vi "ClearResources.vi"() -> ()   [LabVIEW 2020, in "AIM664LV.lvlib"]
uses:
  AIM664LV.lvlib
panel:
  out "resources":T1(array[cluster])
  out "error out":errorcluster
  out "NuOfServers":u32
  out "size(s)":i32
  out "Array":errorcluster[](array[cluster])
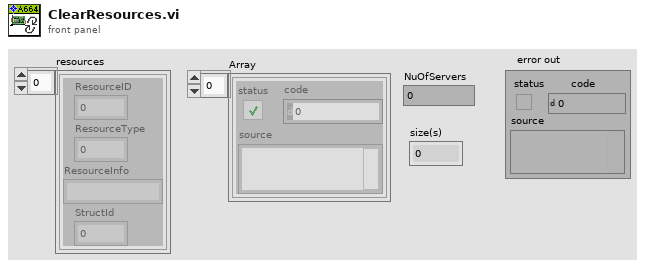
[diagram p1: front panel]
types:
  T1 = cluster{"ResourceID":u32, "ResourceType":u32, "ResourceInfo":string, "StructId":u32}[]
  T2 = cluster{"ResourceID":u32, "ResourceType":u32, "ResourceInfo":string, "StructId":u32}
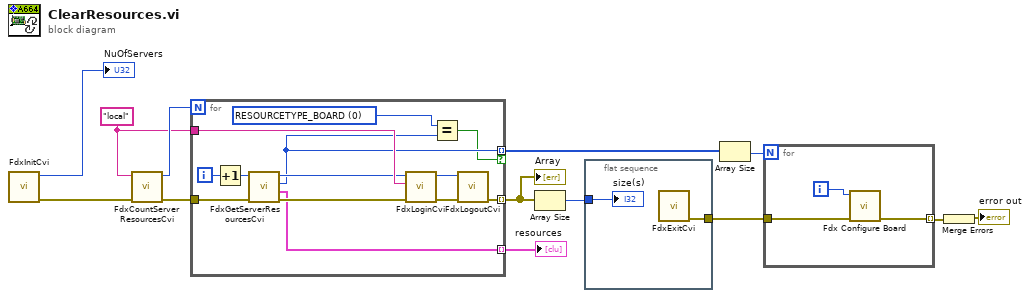
[diagram p0: block diagram]
diagram:
  w6 = "local" ("SrvName(local)")
  n1 = call "FdxInitCvi.vi"() -> ("error out"=w9:errorcluster, "Number of Servers"=→"NuOfServers":u32)  [unwired: 10 in]
  n2 = call "FdxCountServerResourcesCvi.vi"("error in"=w9, "SrvName (local)"=w6) -> ("error out"=w12:errorcluster, "Number of Resources"=w13:u32)  [unwired: 8 in]
  n3 = for {
    N: w13 -> [_]
    tunnel: w12 -> [w26]
    tunnel: [w20] -> w11 mode=indexing
    tunnel: [w19] -> w7 mode=indexing
    tunnel: w6 -> [w18]
    tunnel: [w15] -> w5 mode=indexing if=w14
    i -> [w25]
    w16 = u32 0 items=["RESOURCETYPE_BOARD"=0, "RESOURCETYPE_PORT"=1, "RESOURCETYPE_ALL"=20] ("ResourceType")
    n4 = Increment(x=w25) -> (x+1=w24:i32)
    n5 = call "FdxGetServerResourcesCvi.vi"("error in"=w26, "ServerRElement"=w24) -> ("error out"=w23:errorcluster, "ServerResourceInfo"=w19:T2, "ResourceType"=w15:u32, "Resource ID"=w17:u32)  [unwired: 4 in, 2 out]
    n6 = call "FdxLoginCvi.vi"("error in"=w23, "SrvName"=w18, "ResourceID"=w17) -> ("error out"=w22:errorcluster, "InstrumentHandle"=w21:u32)  [unwired: 7 in]
    n7 = Equal?(x=w16, y=w15) -> (x = y?=w14:bool)
    n8 = call "FdxLogoutCvi.vi"("error in"=w22, "InstrumentHandle"=w21) -> ("error out"=w20:errorcluster)  [unwired: 9 in]
  }
  "Array" <- w11
  "resources" <- w7
  n9 = Array Size(array=w11) -> (size(s)=w10:i32)
  n10 = flat-sequence {
    tunnel: w10 -> [w28]
    tunnel: [w27] -> w3
    frame #0 {
      n11 = call "FdxExitCvi.vi"() -> ("error out"=w27:errorcluster)  [unwired: 11 in]
      "size(s)" <- w28
    }
  }
  n12 = Array Size(array=w5) -> (size(s)=w4:i32)
  n13 = for {
    N: w4 -> [_]
    tunnel: [w30] -> w1 mode=indexing
    tunnel: w3 -> [w29]
    i -> [w31]
    n14 = call "Fdx Configure Board.vi"("error in (no error)"=w29, "board index"=w31) -> ("error out"=w30:errorcluster)  [unwired: 5 in, 4 out]
  }
  n15 = Merge Errors(w1) -> (→"error out":errorcluster)
